vi "Display Input (I32) Popup (Custom).vi"(4 "Message Size":T1={"Message Height"=-1, "Message Width"=-1, "Message Location"=enum."Bottom"} {"Message Width" min=-1 step=1; "Message Height" min=-1 step=1}, 6 "Theme":refnum<class "Theme.lvclass">, 8 "Error In":errorcluster, 9 "Default Input":i32, 10 "Message":string, 11 "Graphic":path) -> (0 "Error Out":errorcluster, 1 "Input Value":i32)   [LabVIEW 2021, in "Pop-Up.lvlib" / "Custom - Input (I32).lvclass"]
doc: "The input (I32) popup will display information to the user and wait for the operator to enter a value and click the button.\n\n<b>Note:</b> This popup type allows the user to define a custom image for the display. The developer should test all settings prior to deployment to make sure that all images and text fit on the screen correctly.\n\n<b>Note:</b> The function <b>Close Pop-Up (I32).vi</b> can be used to send a value when closing this dialog. Otherwise, use Close Pop-Up.vi to close it early.\n\nInputs: +\n-Graphic [path] - path to the image file to display +\n-Message [String] - String Variable to populate Display with +\n-Theme [lvclass] - the theme for the style of the popup +\n-Message Info [typedef enum] +\n -Message Height [I32] - the height for the message text box (-1 = match height of image) +\n -Message Width [I32] - the width for the message text box (-1 = match height of image) +\n -Message Location [Ring] - the location of the image relative to the message text box (left,\n right,bottom, top) +\n-Default Input [I32] - default value for the prompt +\n\nOutputs: +\n-InputValue [I32] - the user's input data\n\n<b>Code Developed By:</b> +\nDaniel Coons +\nhttps://github.com/danielcoons/tsc-pop-up"
uses:
  Custom - Input (I32).lvclass
  Theme/Theme.lvclass
  Popup/message info--typedef.ctl
  Custom - Input (I32).lvclass/Custom - Input (I32).ctl
  Popup/Popup.lvclass
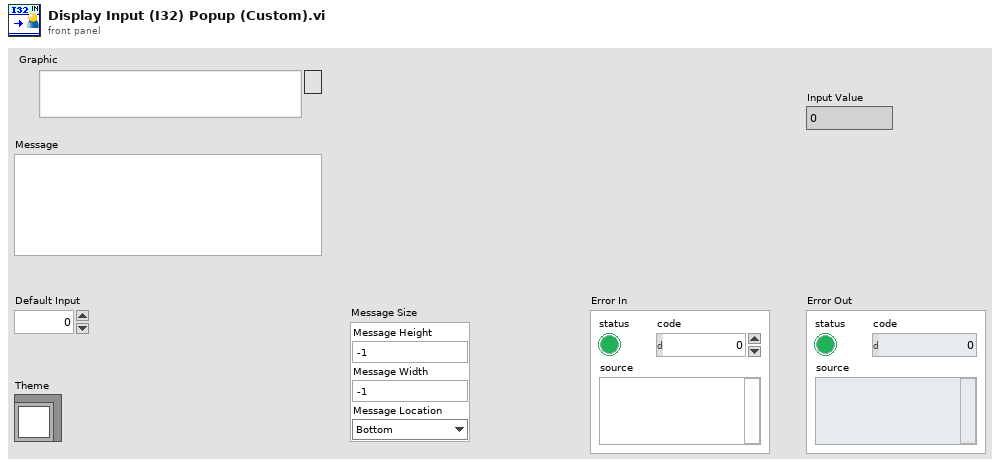
[diagram p1: front panel]
types:
  T1 = typedef "Pop-Up.lvlib/Popup.lvclass/message info--typedef.ctl" = cluster{"Message Height":i32, "Message Width":i32, "Message Location":enum16{"Top", "Bottom", "Right", "Left"}}
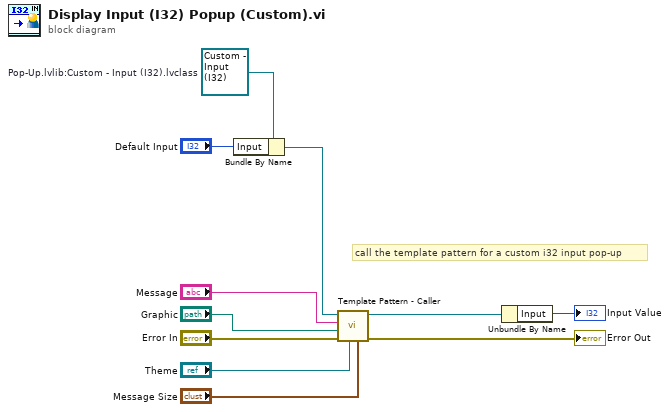
[diagram p0: block diagram]
diagram:
  w6 = refnum<class "Custom - Input (I32).lvclass"> refnum  # Pop-Up.lvlib:Custom - Input (I32).lvclass
  # "call the template pattern for a custom i32 input pop-up"
  n1 = Bundle By Name(cluster=w6, "Input"="Default Input") -> (w5:refnum<class "Custom - Input (I32).lvclass">)
  n2 = call-dynamic "Template Pattern - Caller.vi"("Message Size"="Message Size", "Theme"="Theme", "error in (no error)"="Error In", "Graphic"="Graphic", "Message"="Message", "Pop-Up in"=w5) -> ("error out"=→"Error Out":errorcluster, "Pop-Up out"=w4:refnum<class "Custom - Input (I32).lvclass">)  [unwired: 4 in]
  n3 = Unbundle By Name(w4) -> ("Input"=→"Input Value":i32)
